vi "Read Mode.vi"(8 "error in (no error)":errorcluster, 11 "Pound in":refnum<class "Pound.lvclass">) -> (0 "error out":errorcluster, 2 "Mode":enum16{"Running", "Shutdown"}(ring), 3 "Pound out":refnum<class "Pound.lvclass">)   [LabVIEW 2017, in "Pound.lvclass"]
uses:
  <vilib>/NI/Software Watchdog/Pound/Pound.lvclass
  <vilib>/NI/Software Watchdog/Pound/Pound.lvclass/Pound.ctl
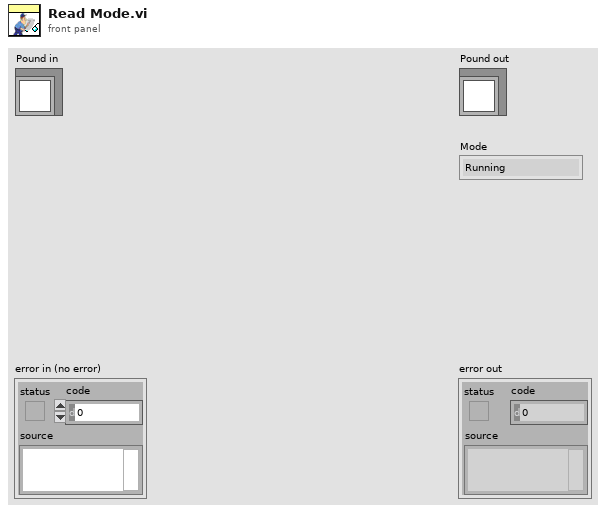
[diagram p1: front panel]
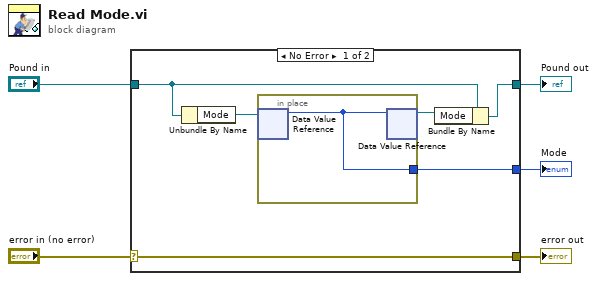
[diagram p0: block diagram]
diagram:
  n1 = case shown="No Error" "error in (no error)" {
    selector: "error in (no error)" -> [w11 w13]
    tunnel: [w11 w13] -> w4
    tunnel: [w9 w14] -> w2
    tunnel: "Pound in" -> [w10 w14]
    tunnel: [w6 _] -> w1
    frame No Error {
      n2 = Unbundle By Name(w10) -> ("Mode"=w8:refnum<data-value>)
      n3 = in-place {
        in-place-border: [w12] -> w6
        n4 = in-place-dvr #1(w8) -> (w12:enum16{"Running", "Shutdown"})  [unwired: 1 out]
        n5 = in-place-dvr #1(w12) -> (w7:refnum<data-value>)  [unwired: 1 out]
      }
      n6 = Bundle By Name(cluster=w10, "Mode"=w7) -> (w9:refnum<class "Pound.lvclass">)
    }
    frame Error {
    }
  }
  "error out" <- w4
  "Pound out" <- w2
  "Mode" <- w1
